vi "MC core logic.vi"(0 "AOL_ref_scan_next":bool, 2 "Trigger pulse (pos. edge)":bool, 5 "Reset_ref_counter":bool, 7 "State":T1=enum."Wait N after Trigger", 9 "Ref count reset enabled":bool, 11 "Ref Scan Cycles":i32, 12 "Acquire MC":bool, 13 "MC":bool) -> (4 "start_aol_ref_scan":bool, 6 "start_ref_scan":bool)   [LabVIEW 2020]
uses:
  FPGA Typedefs/Image State.ctl
  FPGA Typedefs/aol_scan_state.ctl
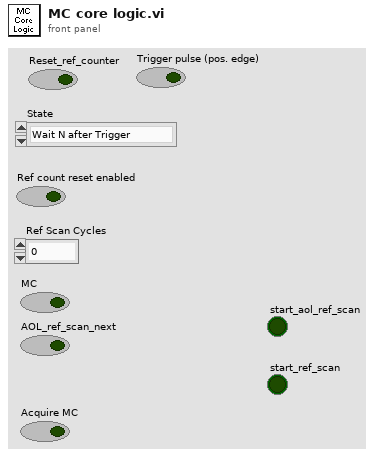
[diagram p1: front panel]
types:
  T1 = typedef "Image State.ctl" = enum16{"Start Up", "Wait for Trigger", "Wait N after Trigger", "DAQ Pointing", "DAQ Scan", "Reference Scan", "Pointing AOL Fill", "Scan AOL FILL", "Reference AOL Fill"}
  T2 = typedef "aol_scan_state.ctl" = enum16{"wait_for_ref_pulse", "signal_aol_ref_scan", "aol_next_scan"}
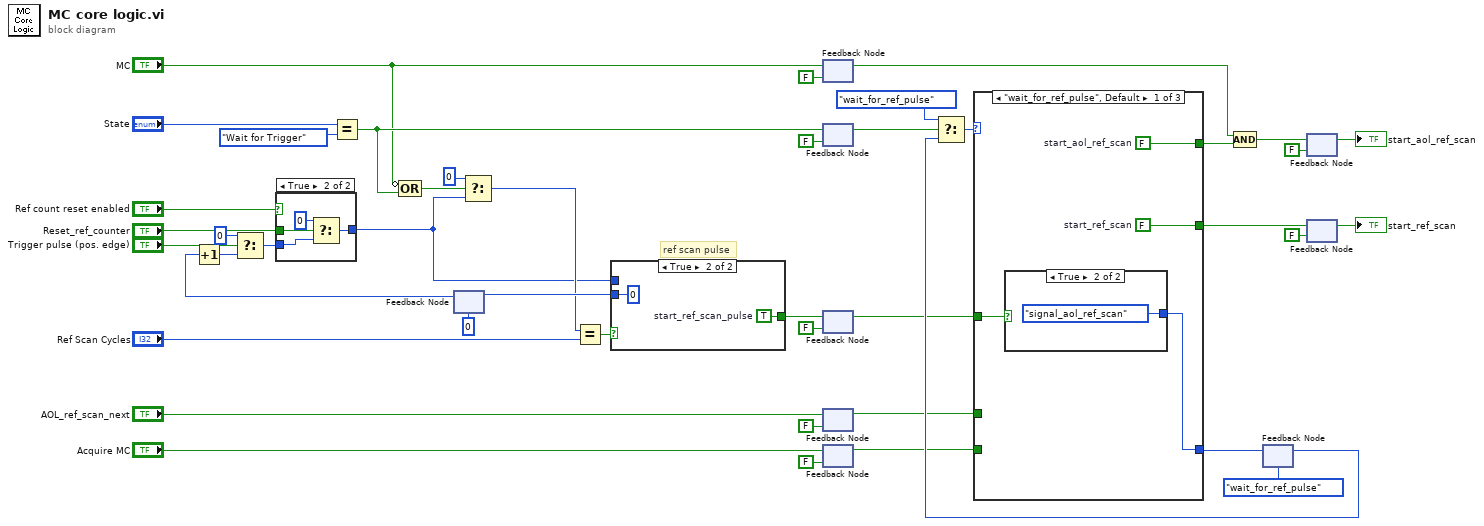
[diagram p0: block diagram]
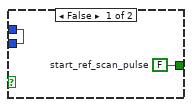
[diagram p3: hidden frame]
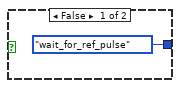
[diagram p4: hidden frame]
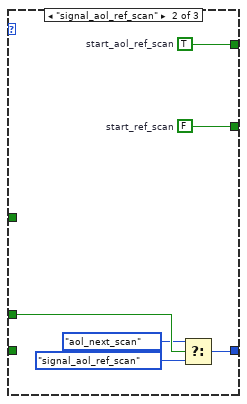
[diagram p5: hidden frame]
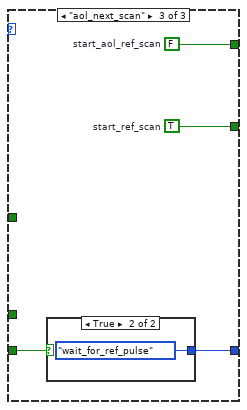
[diagram p6: hidden frame]
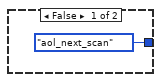
[diagram p7: hidden frame]
diagram:
  # "ref scan pulse"
  n1 = Equal?(x="State", y=Image_State."Wait for Trigger" ("Enum")) -> (x = y?=w21:bool)
  n2 = Compound Arithmetic op=OR(invert "MC", w21) -> (w31:bool)
  n3 = feedback #1(0) -> (w27:i32)
  n4 = Increment(x=w27) -> (x+1=w26:i32)
  n5 = Select(t=0, s="Trigger pulse (pos. edge)", f=w26) -> (s? t:f=w29:i32)
  n6 = case shown="True" "Ref count reset enabled" {
    tunnel: [w45 w48] -> w25
    tunnel: w29 -> [w45 w47]
    tunnel: "Reset_ref_counter" -> [_ w46]
    frame False {
    }
    frame True {
      n7 = Select(t=0, s=w46, f=w47) -> (s? t:f=w48:i32)
    }
  }
  n8 = Select(t=0, s=w31, f=w25) -> (s? t:f=w30:i32)
  n9 = Equal?(x=w30, y="Ref Scan Cycles") -> (x = y?=w32:bool)
  n10 = case shown="True" w32 {
    tunnel: w25 -> [w50 _]
    tunnel: [w51 w53] -> w18
    tunnel: [w50 0] -> w36
    frame False {
      w51 = FALSE  # start_ref_scan_pulse
    }
    frame True {
      w53 = TRUE  # start_ref_scan_pulse
    }
  }
  n11 = feedback-in #1(w36) -> ()
  n12 = feedback-in #2("MC") -> ()
  n13 = feedback #2(FALSE ("MC")) -> (w10:bool)
  n14 = feedback-in #3(w21) -> ()
  n15 = feedback #3(FALSE) -> (w2:bool)
  n16 = feedback-in #4(w18) -> ()
  n17 = feedback #4(FALSE ("start_ref_scan_pulse")) -> (w4:bool)
  n18 = feedback-in #5("AOL_ref_scan_next") -> ()
  n19 = feedback #5(FALSE ("AOL_ref_scan_next")) -> (w8:bool)
  n20 = feedback-in #6("Acquire MC") -> ()
  n21 = feedback #6(FALSE ("Acquire MC")) -> (w6:bool)
  n22 = feedback #7(aol_scan_state."wait_for_ref_pulse") -> (w38:T2)
  n23 = Select(t=aol_scan_state."wait_for_ref_pulse", s=w2, f=w38) -> (s? t:f=w44:T2)
  n24 = case shown="\"wait_for_ref_pulse\", Default" w44 {
    tunnel: [w57 w60 w68] -> w39
    tunnel: w8 -> [_ w63 _]
    tunnel: w4 -> [w54 _ _]
    tunnel: [w56 w64 w66] -> w42
    tunnel: w6 -> [_ _ w69]
    tunnel: [w55 w65 w67] -> w19
    frame "wait_for_ref_pulse", Default {
      w55 = FALSE  # start_ref_scan
      w56 = FALSE  # start_aol_ref_scan
      n25 = case shown="True" w54 {
        tunnel: [aol_scan_state."wait_for_ref_pulse" aol_scan_state."signal_aol_ref_scan"] -> w57
        frame False {
        }
        frame True {
        }
      }
    }
    frame "signal_aol_ref_scan" {
      w65 = FALSE  # start_ref_scan
      w64 = TRUE  # start_aol_ref_scan
      n26 = Select(t=aol_scan_state."aol_next_scan", s=w63, f=aol_scan_state."signal_aol_ref_scan") -> (s? t:f=w60:T2)
    }
    frame "aol_next_scan" {
      w67 = TRUE  # start_ref_scan
      w66 = FALSE  # start_aol_ref_scan
      n27 = case shown="True" w69 {
        tunnel: [aol_scan_state."aol_next_scan" aol_scan_state."wait_for_ref_pulse"] -> w68
        frame False {
        }
        frame True {
        }
      }
    }
  }
  n28 = Compound Arithmetic op=AND(w10, w42) -> (w20:bool)
  n29 = feedback-in #7(w39) -> ()
  n30 = feedback-in #8(w20) -> ()
  n31 = feedback #8(FALSE ("MC")) -> (→"start_aol_ref_scan":bool)
  n32 = feedback-in #9(w19) -> ()
  n33 = feedback #9(FALSE ("MC")) -> (→"start_ref_scan":bool)
